vi "Query the Test Parameters for MANU.vi"(8 "error in":errorcluster, 10 "Manual test number of test parameters":u8 max=100, 11 "VISA resource name":refnum<visa-resource-name>) -> (0 "error out":errorcluster, 1 "Return the count of Test Parameters String":u16, 2 "Return the Test Parameters String":string, 3 "VISA resource name out":refnum<visa-resource-name>)   [LabVIEW 2011, in "GPT-9000.lvlib"]
uses:
  <instrlib>/GPT-9000/GPT-9000.lvlib
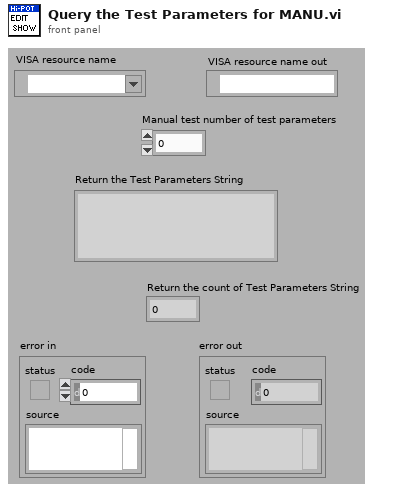
[diagram p1: front panel]
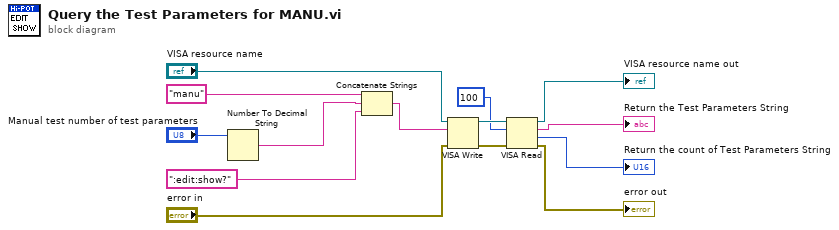
[diagram p0: block diagram]
diagram:
  n1 = Number To Decimal String(number="Manual test number of test parameters") -> (decimal integer string=w12:string)  [unwired: 1 in]
  n2 = Concatenate Strings("manu", w12, ":edit:show?") -> (w8:string)
  n3 = VISA Write(VISA resource name="VISA resource name", write buffer=w8, error in (no error)="error in") -> (VISA resource name out=w6:refnum<visa-resource-name>, error out=w7:errorcluster)  [unwired: 1 out]
  n4 = VISA Read(VISA resource name=w6, byte count=u32 100, error in (no error)=w7) -> (VISA resource name out=→"VISA resource name out":refnum<visa-resource-name>, read buffer=→"Return the Test Parameters String":string, return count=→"Return the count of Test Parameters String":u32, error out=→"error out":errorcluster)
